vi "update-bit-payload-by-tag.vi"(0 "CANtable in":refnum<class "bAPPdata.lvclass">, 5 "frame.tag":string, 7 "Array":bool[](array[boolean]), 9 "start.pos":i32, 11 "error in (no error)":errorcluster) -> (4 "CANtable out":refnum<class "bAPPdata.lvclass">, 15 "error out":errorcluster)   [LabVIEW 2015, in "bAPPdata.lvclass"]
uses:
  bAPPdata.lvclass
  bAPPdata.lvclass/bAPPdata.ctl
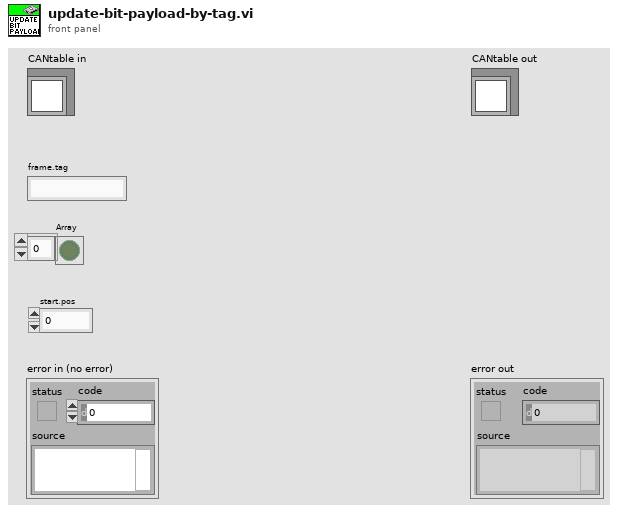
[diagram p1: front panel]
types:
  T1 = typedef "bAPPdata.lvclass/table-data.ctl" = T2[]
  T2 = typedef "bAPPdata.lvclass/table-contents.ctl" = cluster{"id":u32, "tag":string, "frame.type":T3, "last.frame":T4, "tMsgData":T6, "child.tags":string[], "bit-payload":bool[]}
  T3 = typedef "frame.type.ctl" = enum16{"FRAME NOT DEFINED", "DUT OUTPUT FRAME", "DUT INPUT FRAME"}
  T4 = typedef "XNET Frame CAN.ctl" = cluster{"timestamp":timestamp, "payload":u8[], "identifier":u32, "type":T5, "extended?":bool, "echo?":bool}
  T5 = typedef "XNET Frame Type CAN.ctl" = u8
  T6 = typedef "nMsgData.ctl" = cluster{"dwID":u32, "count":u32, "dwCycleTime":dbl, "dwTime":dbl, "new msg":bool}
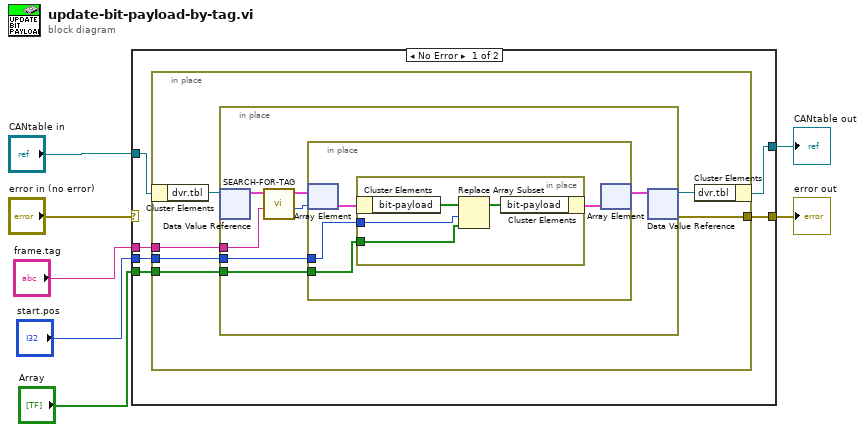
[diagram p0: block diagram]
diagram:
  n1 = case shown="No Error" "error in (no error)" {
    selector: "error in (no error)" -> [_ w36]
    tunnel: [w11 w36] -> w6
    tunnel: [w12 w35] -> w4
    tunnel: "CANtable in" -> [w13 w35]
    tunnel: "frame.tag" -> [w10 _]
    tunnel: "Array" -> [w9 _]
    tunnel: "start.pos" -> [w8 _]
    frame No Error {
      n2 = in-place {
        in-place-border: [w17] -> w11
        in-place-border: w10 -> [w16]
        in-place-border: w9 -> [w15]
        in-place-border: w8 -> [w14]
        n3 = in-place-cluster #1(w13) -> ("dvr.tbl"=w19:refnum<data-value>)
        n4 = in-place {
          in-place-border: w16 -> [w25]
          in-place-border: w15 -> [w21]
          in-place-border: w14 -> [w20]
          n5 = in-place-dvr #2(w19) -> (w26:T1)  [unwired: 1 out]
          n6 = call "SEARCH-FOR-TAG.vi"("tag"=w25, "tbl.list"=w26) -> ("idx"=w23:i32, "tbl.list out"=w24:T2[])  [unwired: 8 in]
          n7 = in-place {
            in-place-border: w21 -> [w28]
            in-place-border: w20 -> [w27]
            n8 = in-place-array #3(w24, w23) -> (w30:T2)
            n9 = in-place {
              in-place-border: w28 -> [w32]
              in-place-border: w27 -> [w31]
              n10 = in-place-cluster #4(w30) -> ("bit-payload"=w34:bool[])
              n11 = Replace Array Subset(array=w34, new element=w32, index=w31) -> (w33:bool[])
              n12 = in-place-cluster #4("bit-payload"=w33) -> (w29:T2)
            }
            n13 = in-place-array #3(w29) -> (w22:T2[])  [unwired: 1 out]
          }
          n14 = in-place-dvr #2(w22) -> (w18:refnum<data-value>, w17:errorcluster)
        }
        n15 = in-place-cluster #1("dvr.tbl"=w18) -> (w12:refnum<class "bAPPdata.lvclass">)
      }
    }
    frame Error {
    }
  }
  "error out" <- w6
  "CANtable out" <- w4
